vi "WPI_SimpleGyroFGV.vi"(0 "SimpleGyroDevRef":T1, 1 "Operation":enum16{"set", "get"}(ring), 5 "Reset":bool, 7 "Calibrated":bool, 9 "Angle":dbl, 11 "Rate":dbl) -> (4 "SimpleGyroDevRef":T1, 6 "Reset?":bool, 8 "Calibrated?":bool, 10 "Angle":dbl, 15 "Rate":dbl)   [LabVIEW 2014, in "SimpleGyro.lvlib"]
uses:
  SimpleGyro.lvlib
  WPI_SimpleGyroDevRef.ctl
  <vilib>/Rock Robotics/SystemInterfaces/Typedef/FPGA_TypedefDigitalModule.ctl
  <vilib>/Rock Robotics/SystemInterfaces/spilib/spi_bus.ctl
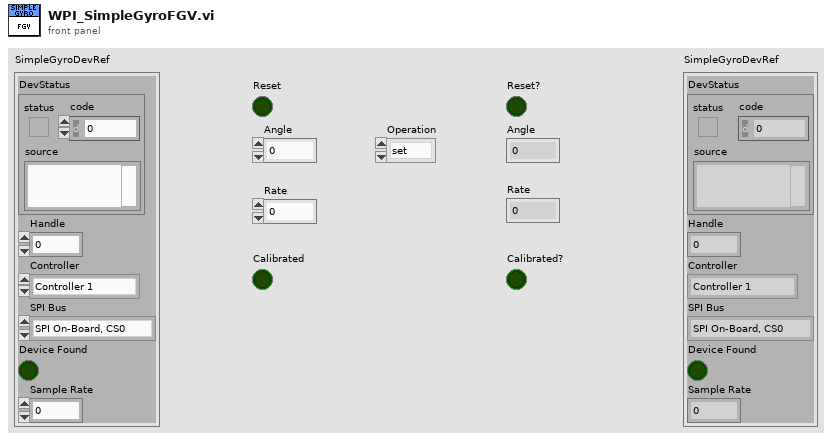
[diagram p1: front panel]
types:
  T1 = typedef "SimpleGyro.lvlib/WPI_SimpleGyroDevRef.ctl" = cluster{"DevStatus":errorcluster, "Handle":i32, "Controller":T2, "SPI Bus":T3, "Device Found":bool, "Sample Rate":dbl}
  T2 = typedef "FPGA_TypedefDigitalModule.ctl" = enum16{"Controller 1"}
  T3 = typedef "spi_bus.ctl" = enum16{"SPI On-Board, CS0", "SPI On-Board, CS1", "SPI On-Board, CS2", "SPI On-Board, CS3", "SPI MXP", "Invalid"}
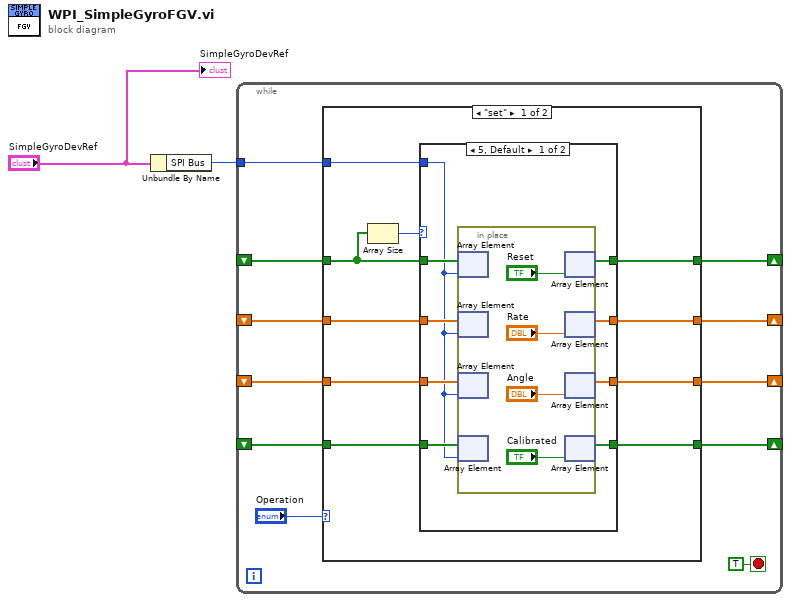
[diagram p0: block diagram]
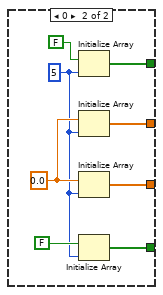
[diagram p2: hidden frame]
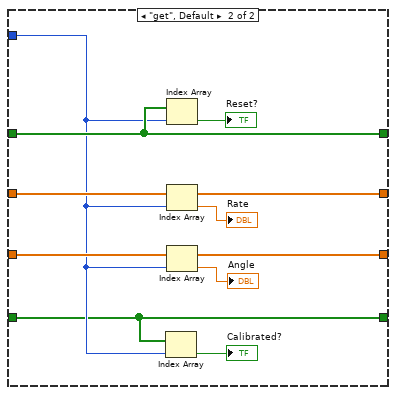
[diagram p3: hidden frame]
diagram:
  n1 = Unbundle By Name("SimpleGyroDevRef") -> ("SPI Bus"=w2:T3)
  n2 = while {
    tunnel: w2 -> [w7]
    shift-right: [w11] -> _
    shift-left: _ -> [w9]
    shift-right: [w10] -> _
    shift-left: _ -> [w8]
    shift-right: [w6] -> _
    shift-left: _ -> [w5]
    shift-right: [w4] -> _
    shift-left: _ -> [w3]
    stop <- TRUE stop-if-true
    n3 = case shown="\"set\"" "Operation" {
      tunnel: [w23 w53] -> w11
      tunnel: [w22 w52] -> w10
      tunnel: w9 -> [w20 w53]
      tunnel: w8 -> [w19 w52]
      tunnel: w7 -> [w18 w46]
      tunnel: [w17 w49] -> w6
      tunnel: w5 -> [w16 w49]
      tunnel: [w15 w45] -> w4
      tunnel: w3 -> [w14 w45]
      frame "set" {
        n4 = Array Size(array=w20) -> (size(s)=w21:i32)
        n5 = case shown="5, Default" w21 {
          tunnel: [w30 w43] -> w23
          tunnel: [w29 w42] -> w22
          tunnel: w20 -> [w32 _]
          tunnel: w19 -> [w31 _]
          tunnel: w18 -> [w24 _]
          tunnel: [w27 w41] -> w17
          tunnel: w16 -> [w28 _]
          tunnel: [w26 w37] -> w15
          tunnel: w14 -> [w25 _]
          frame 5, Default {
            n6 = in-place {
              n7 = in-place-array #1(w32, w24) -> ()  [unwired: 1 out]
              n8 = in-place-array #2(w28, w24) -> ()  [unwired: 1 out]
              n9 = in-place-array #3(w31, w24) -> ()  [unwired: 1 out]
              n10 = in-place-array #4(w25, w24) -> ()  [unwired: 1 out]
              n11 = in-place-array #1("Reset") -> (w30:bool[])  [unwired: 1 out]
              n12 = in-place-array #2("Rate") -> (w27:dbl[])  [unwired: 1 out]
              n13 = in-place-array #3("Angle") -> (w29:dbl[])  [unwired: 1 out]
              n14 = in-place-array #4("Calibrated") -> (w26:bool[])  [unwired: 1 out]
            }
          }
          frame 0 {
            w40 = 0.0 ("Angle")
            w38 = 5 ("dimension size")
            n15 = Initialize Array(FALSE ("Reset"), w38) -> (w43:bool[])
            n16 = Initialize Array(w40, w38) -> (w41:dbl[])
            n17 = Initialize Array(w40, w38) -> (w42:dbl[])
            n18 = Initialize Array(FALSE, w38) -> (w37:bool[])
          }
        }
      }
      frame "get", Default {
        n19 = Index Array(array=w45, index=w46) -> (element=→"Calibrated?":bool)
        n20 = Index Array(array=w53, index=w46) -> (element=→"Reset?":bool)
        n21 = Index Array(array=w49, index=w46) -> (element=→"Rate":dbl)
        n22 = Index Array(array=w52, index=w46) -> (element=→"Angle":dbl)
      }
    }
  }
  "SimpleGyroDevRef" <- "SimpleGyroDevRef"
